vi "Apply best shape.vi"(8 "error in (no error)":errorcluster, 11 "RSA in":refnum<class "RSA.lvclass">) -> (0 "error out":errorcluster, 3 "RSA out":refnum<class "RSA.lvclass">)   [LabVIEW 2012, in "RSA.lvclass"]
uses:
  RSA.lvclass
  RSA.lvclass/RSA.ctl
  <vilib>/Distrio/Murmex/Murmex/Murmex.lvclass
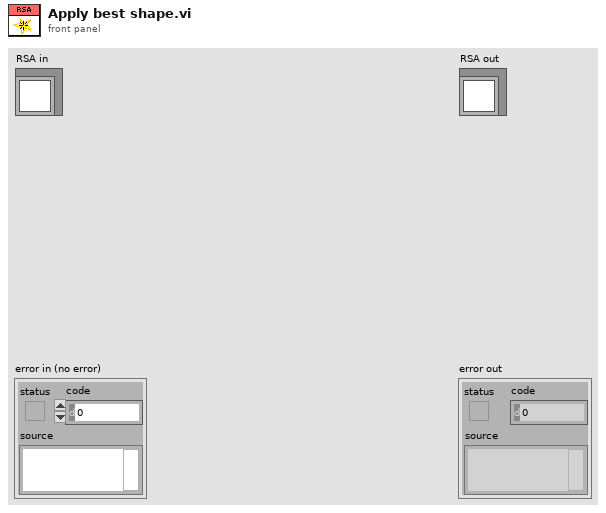
[diagram p1: front panel]
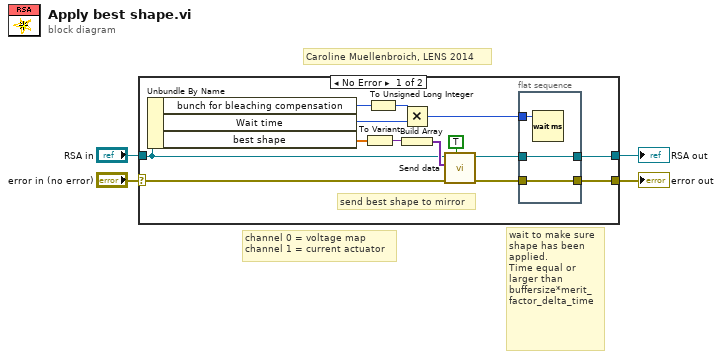
[diagram p0: block diagram]
diagram:
  # "wait to make sure shape has been applied.\nTime equal or larger than buffersize*merit_factor_delta_time"
  # "channel 0 = voltage map\nchannel 1 = current actuator"
  # "Caroline Muellenbroich, LENS 2014"
  n1 = case shown="No Error" "error in (no error)" {
    selector: "error in (no error)" -> [w10 w23]
    tunnel: [w9 w23] -> w3
    tunnel: [w11 w22] -> w1
    tunnel: "RSA in" -> [w12 w22]
    frame No Error {
      # "send best shape to mirror"
      n2 = Unbundle By Name(w12) -> ("bunch for bleaching compensation"=w7:i32, "Wait time"=w8:u32, "best shape"=w13:dbl[])
      n3 = To Variant(anything=w13) -> (Variant=w18:variant)
      n4 = To Unsigned Long Integer(number=w7) -> (unsigned 32bit integer=w5:u32)
      n5 = Multiply(x=w5, y=w8) -> (x*y=w6:u32)
      n6 = Build Array(w18) -> (w17:variant[])
      n7 = call <vilib>:"Send data.vi"("is finalised data? (T)"=TRUE, "error in (no error)"=w10, "data (channels array)"=w17, "Murmex in"=w12) -> ("error out"=w14:errorcluster, "Murmex out"=w15:refnum<class "RSA.lvclass">)  [unwired: 6 in]
      n8 = flat-sequence {
        tunnel: w15 -> [w21]
        tunnel: [w21] -> w11
        tunnel: w14 -> [w20]
        tunnel: [w20] -> w9
        tunnel: w6 -> [w19]
        frame #0 {
          n9 = Wait (ms)(milliseconds to wait=w19) -> ()  [unwired: 1 out]
        }
      }
    }
    frame Error {
    }
  }
  "error out" <- w3
  "RSA out" <- w1
